vi "Set Velocity.vi"(8 "error in (no error)":errorcluster, 10 "Velocity":u16, 11 "Serial Controller in":refnum<class "Serial Controller.lvclass">) -> (0 "error out":errorcluster, 3 "Serial Controller out":refnum<class "Serial Controller.lvclass">)   [LabVIEW 2014, in "Serial Controller.lvclass"]
uses:
  Serial Controller.lvclass
  Serial Controller.lvclass/Serial Controller.ctl
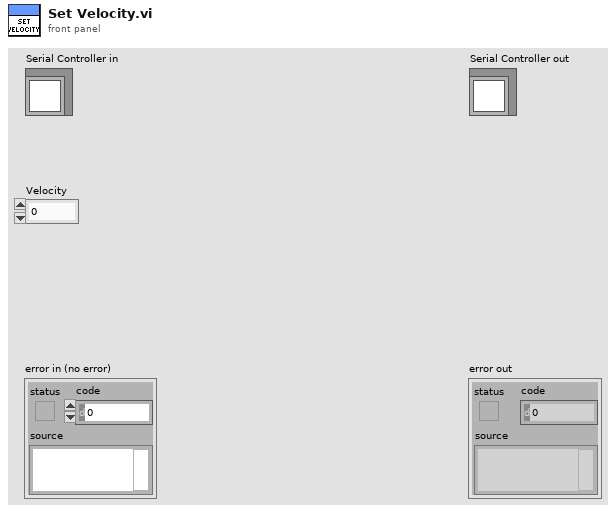
[diagram p1: front panel]
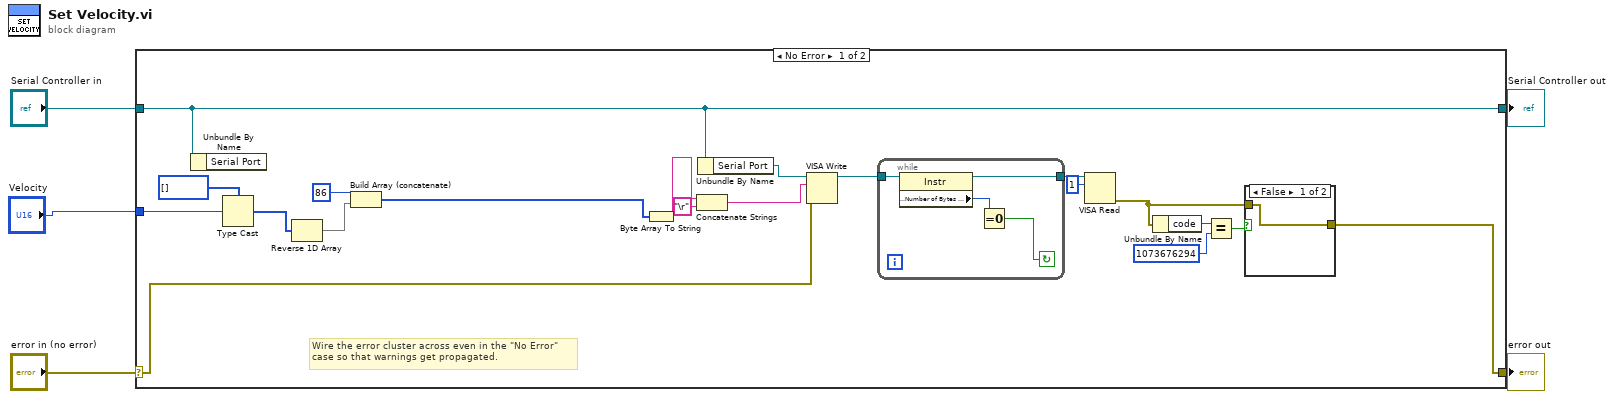
[diagram p0: block diagram]
diagram:
  n1 = case shown="No Error" "error in (no error)" {
    selector: "error in (no error)" -> [w9 w32]
    tunnel: [w8 w32] -> w4
    tunnel: [w10 w31] -> w2
    tunnel: "Serial Controller in" -> [w10 w31]
    tunnel: "Velocity" -> [w25 _]
    frame No Error {
      # "Wire the error cluster across even in the \"No Error\"\ncase so that warnings get propagated."
      n2 = Unbundle By Name(w10) -> ()  [unwired: 1 out]
      n3 = Type Cast(type=u8[] [], x=w25) -> (*(type *) &x=w7:u8[])
      n4 = Reverse 1D Array(array=w7) -> (reversed array=w6:u8[])
      n5 = Build Array (concatenate)(u8 86, w6) -> (w11:u8[])
      n6 = Byte Array To String(unsigned byte array=w11) -> (string=w22:string)
      n7 = Concatenate Strings(w22, "\r" ("string")) -> (w19:string)
      n8 = Unbundle By Name(w10) -> ("Serial Port"=w20:refnum<visa-resource-name>)
      n9 = VISA Write(VISA resource name=w20, write buffer=w19, error in (no error)=w9) -> (VISA resource name out=w18:refnum<visa-resource-name>)  [unwired: 2 out]
      n10 = while {
        tunnel: w18 -> [w30]
        tunnel: [w28] -> w17
        stop <- w27 continue-if-true
        n11 = property class="Instr"(reference=w30) -> (reference out=w28:refnum<visa-resource-name>, "Serial Settings:Number of Bytes at Serial Port"=w29:u32)  [unwired: 1 in, 1 out]
        n12 = Equal To 0?(x=w29) -> (x = 0?=w27:bool)
      }
      n13 = VISA Read(VISA resource name=w17, byte count=u32 1) -> (error out=w12:errorcluster)  [unwired: 1 in, 3 out]
      n14 = Unbundle By Name(w12) -> ("code"=w15:i32)
      n15 = Equal?(x=w15, y=1073676294) -> (x = y?=w13:bool)
      n16 = case shown="False" w13 {
        tunnel: w12 -> [w26 _]
        tunnel: [w26 _] -> w8
        frame False {
        }
        frame True {
        }
      }
    }
    frame Error {
    }
  }
  "error out" <- w4
  "Serial Controller out" <- w2
